vi "Write Attribute.vi"(8 "error in (no error)":errorcluster, 10 "Attribute":T1, 11 "Attribute-XML in":refnum<class "Attribute-XML.lvclass">) -> (0 "error out":errorcluster, 3 "Attribute-XML out":refnum<class "Attribute-XML.lvclass">)   [LabVIEW 2013, in "HardwareCharacterization.lvlib" / "Attribute-XML.lvclass"]
uses:
  Attribute-XML.lvclass
  Attributes.ctl
  Attribute-XML.lvclass/Attribute-XML.ctl
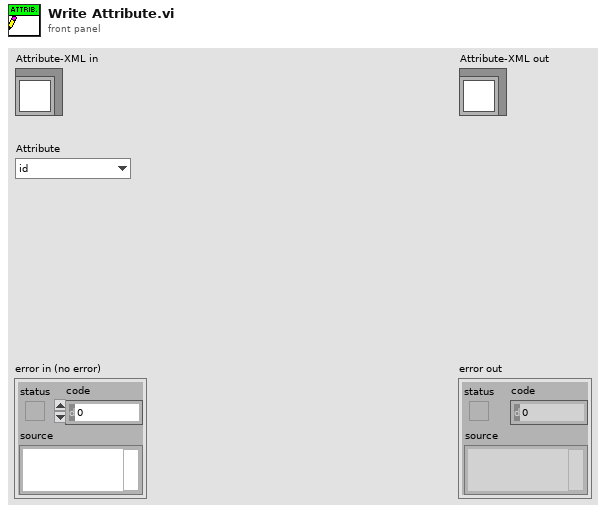
[diagram p1: front panel]
types:
  T1 = typedef "HardwareCharacterization.lvlib/Attribute-XML.lvclass/Attributes.ctl" = enum16{"id"}
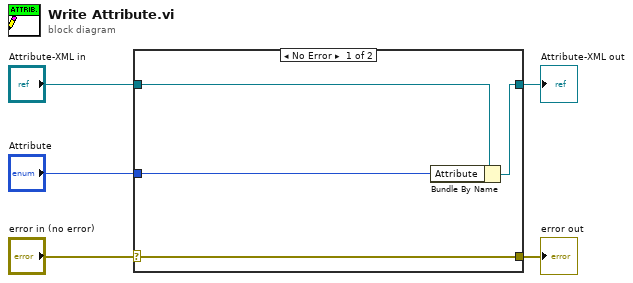
[diagram p0: block diagram]
diagram:
  n1 = case shown="No Error" "error in (no error)" {
    selector: "error in (no error)" -> [w9 w10]
    tunnel: [w9 w10] -> w4
    tunnel: [w7 w11] -> w2
    tunnel: "Attribute-XML in" -> [w8 w11]
    tunnel: "Attribute" -> [w6 _]
    frame No Error {
      n2 = Bundle By Name(cluster=w8, "Attribute"=w6) -> (w7:refnum<class "Attribute-XML.lvclass">)
    }
    frame Error {
    }
  }
  "error out" <- w4
  "Attribute-XML out" <- w2
